vi "struct_ads_piStar_pyxgTM.vi"(0 "Reference working pair (Input)":i64, 1 "Molar fraction of refrigerant in adsorbed phase in mol/mol (Input)":dbl, 2 "Molar fraction of refrigerant in vapor phase in mol/mol (Input)":dbl, 3 "pressure Pa (Input)":dbl, 5 "Temperature in K (Input)":dbl, 7 "Activity coefficient of refrigerant in adsorbed phase (Input)":dbl, 9 "Molar mass of refrigerant M in kg/mol (Input)":dbl, 11 "Error (Input)":errorcluster) -> (4 "Reduced spreading pressure in kg/mol (Output)":dbl, 15 "Error (Output)":errorcluster caption="Error(Output)")   [LabVIEW 2017]
doc: "ads_piStar_pyxgTM:\n * ------------------\n *\n * Calculates reduced spreading pressure piStar in kg/mol depending on\n * equilibrium pressure p in Pa, molar fraction of refrigerant in vapor phase\n * in mol/mol, molar fraction of refrigerant in adsorbed phase in mol/mol,\n * activity coefficient of refrigerant in adsorbed phase, equilibrium\n * temperature T in K and molar mass of refrigerant M in kg/mol. The reduced\n * spreading pressure is defined as follows:\n *\n * piStar = A * pi / (R * T * m_sorbent) = 1 / M *\n * Integral_0^p0{w(p,T) / p * dp}\n *\n * where p0 = p_total*y / (gamma*x)\n *\n * Parameters:\n * -----------\n * double p_total_Pa:\n * Total pressure of vapor phase in Pa.\n * double y_molmol:\n * Molar fraction of refrigerant in vapor phase in mol/mol.\n * double x_molmol:\n * Molar fraction of refrigerant in adsorbed phase in mol/mol.\n * double gamma:\n * Activity coefficient of refrigerant in adsorbed phase.\n * double T_K:\n * Equilibrium temperature in K.\n * double M_kgmol:\n * Molar mass of refrigerant M in kg/mol.\n * struct *WorkingPair:\n * Pointer of WorkingPair-struct.\n *\n * Returns:\n * --------\n * double:\n * Reduced spreading pressure in kg/mol.\n *\n * History:\n * --------\n * 07/13/2021, by Jannik Driesel (supervised by Mirko Engelpracht):\n * First implementation."
uses:
  data/win32bit/libsorpPropLib.dll
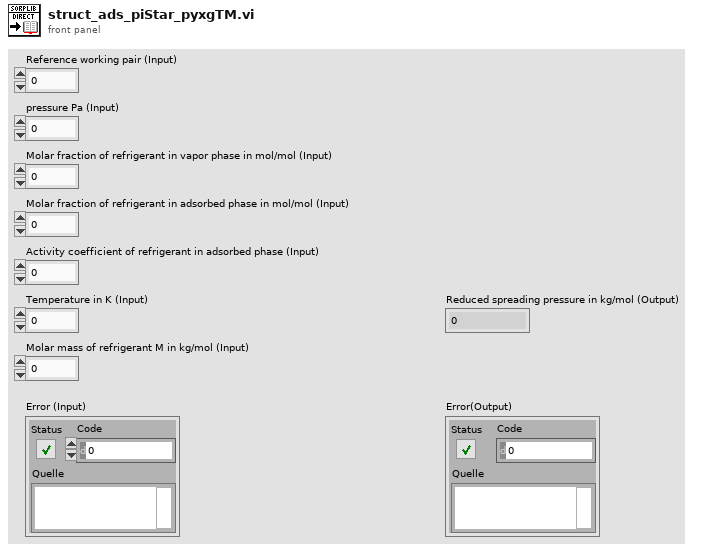
[diagram p1: front panel]
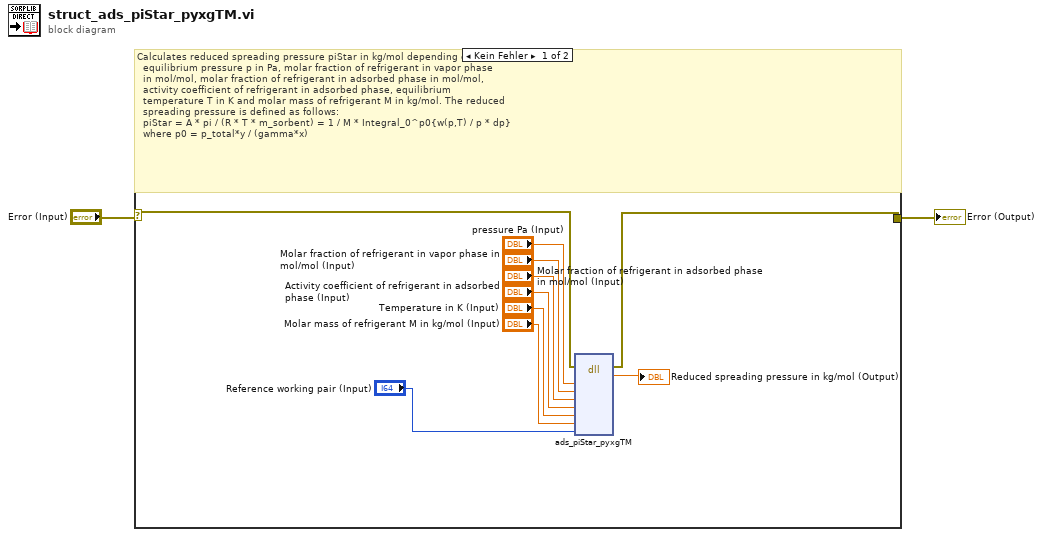
[diagram p0: block diagram]
diagram:
  n1 = case shown="Kein Fehler" "Error (Input)" {
    selector: "Error (Input)" -> [w11 w13]
    tunnel: [w10 w13] -> w1
    frame No Error {
      # "Calculates reduced spreading pressure piStar in kg/mol depending on\n  equilibrium pressure p in Pa, molar fraction of refrigerant in vapor phase\n  in mol/mol, molar fraction of refrigerant in adsorbed phase in mol/mol,\n  activity coefficient of refrigerant in adsorbed phase, equilibrium\n  temperature T in K and molar mass of refrigerant M in kg/mol. The reduced\n  spreading pressure is defined as follows:\n \tpiStar = A * pi / (R * T * m_sorbent) = 1 / M * Integral_0^p0{w(p,T) / p * dp}\n  where p0 = p_total*y / (gamma*x)"
      n2 = dll-call lib="D:/Driesel/SorpLibLocal/LabVIEW_wrapper/data/win32bit/libsorpPropLib.dll" fn="ads_piStar_pyxgTM"(error in=w11, "p_total_Pa"="pressure Pa (Input)", "y_molmol"="Molar fraction of refrigerant in vapor phase in mol/mol (Input)", "x_molmol"="Molar fraction of refrigerant in adsorbed phase in mol/mol (Input)", "gamma"="Activity coefficient of refrigerant in adsorbed phase (Input)", "T_K"="Temperature in K (Input)", "M_kgmol"="Molar mass of refrigerant M in kg/mol (Input)", "workingPair"="Reference working pair (Input)") -> (error out=w10:errorcluster, "piStar_kgmol"=→"Reduced spreading pressure in kg/mol (Output)":dbl)  [unwired: 9 in, 1 out]
    }
    frame Error {
      # "Error - No calculations"
    }
  }
  "Error (Output)" <- w1
